vi "BlackBox.vi"() -> ()   [LabVIEW 2019]
uses:
  <vilib>/Simulation/Scripting/Companion Diagram/SimConfigNode/SimParams.ctl
  <vilib>/Simulation/Scripting/Companion Diagram/SimConfigNode/_simSolvers.ctl
  <vilib>/Simulation/Implementation/Shared/SIMSCR Execution Mode.ctl
  <vilib>/Simulation/Param Hierarchy/Typedefs/SIMPH Param Control Actions.ctl
  <vilib>/DAQmx/read.llb/DAQmx Read (Analog DBL 1Chan 1Samp).vi
  <vilib>/Simulation/Implementation/Shared/NILVSim_ParamChanged.vi
  <vilib>/Simulation/Implementation/Shared/NILVSIM_BeginStep.vi
  <vilib>/Simulation/Implementation/Shared/NILVSim_Manager.vi
  <vilib>/Utility/error.llb/Clear Errors.vi
  <vilib>/Simulation/Implementation/Shared/NILVSim_FinalizeModel.vi
  <vilib>/DAQmx/write.llb/DAQmx Write (Analog DBL 1Chan 1Samp).vi
  <vilib>/DAQmx/miscellaneous.llb/DAQmx Fill In Error Info.vi
  <vilib>/Simulation/Implementation/Shared/SIM Unbundle Sim Info.vi
  <vilib>/Simulation/Implementation/Shared/NILVSim_Initialize.vi
  <vilib>/Simulation/Utility/Implementation/NILVSim Get Time and IsAcceptedStep.vi
  <vilib>/Simulation/Implementation/Shared/SIMSH Read Queue.vi
  <vilib>/Simulation/Implementation/Shared/NILVSim_GetModelError.vi
  <vilib>/Simulation/Implementation/Shared/SIM Bundle Sim Info.vi
  <vilib>/Simulation/Implementation/XNodeFramework/SimXNode/SimX.xnode
  Industry 4-0 lab/Airheater Model subsystem.vi
  <vilib>/Simulation/Scripting/Companion Diagram/SimConfigNode/SimDog.xnode
  <vilib>/Simulation/Implementation/Shared/NI_SIM_Implementation.lvlib
panel:
  in  "stop":bool
  out "Temperature Chart":dbl(graph)
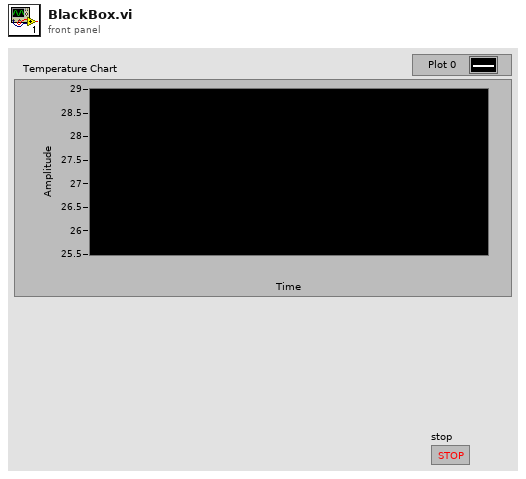
[diagram p1: front panel]
types:
  T1 = enum16{"Simulate to Completion", "Single Time-Step Simulation (Fixed Step Only)"}
  T2 = typedef "SIMSCR Execution Mode.ctl" = enum16{"Simulate to Completion", "Single Time-Step Simulation (Fixed Step Only)"}
  T3 = typedef "SIMPH Param Control Actions.ctl" = enum16{"get params", "set params"}
  T4 = cluster{"SIMSH Sim Time":dbl, "Operand2":dbl, "Multiplication 3":cluster{"Result":dbl}, "Integrator":cluster{"output":dbl}, "Multiplication 2":cluster{"Result":dbl}, "Summation 2":cluster{"Result":dbl}, "Transport Delay":cluster{"output":dbl}, "Summation":cluster{"Result":dbl}, "Multiplication":cluster{"Result":dbl}}
  T5 = typedef "SimParams.ctl" = cluster{"Initial Time (s)":dbl, "Final Time (s)":dbl, "Step Size (s)":dbl, "ODE Solver":T6, "Minimum Step Size (s)":dbl, "Maximum Step Size (s)":dbl, "Relative Tolerance":dbl, "Absolute Tolerance":dbl, "Software Timing":bool, "Initial Step Size (s)":dbl, "Automatic Fixed Step Size?":bool, "Automatic Discrete Step Size?":bool, "Discrete Step Size (s)":dbl, "Calculate using Time Step":bool, "Solver Wired?":bool, "Prev.Frm.Expected End":u64, "Prev.Frm.Actual End":u64, "Prev.Frm.Finished Late?":bool, "Prev.Iter.Expected End":u64, "Prev.Iter.Actual End":u64, "Prev.Iter.Finished Late?":bool, "Expected Iteration Start":u64, "Actual Iteration Start":u64, "Expected Frame Start":u64, "Actual Frame Start":u64, "Source Name":string, "Name":string, "Period":i64, "Deadline":i64, "Offset":i64, "Start":i64, "Priority":i32, "Timeout":i32, "Processor":i32, "Mode":enum32{"No Change", "Process missed periods, maintain original phase", "Discard missed periods, maintain original phase", "Process missed periods, ignore original phase", "Discard missed periods, ignore original phase"}, "Wakeup reason":enum32{"Normal", "Aborted", "Asynchronous wakeup", "Timing source error", "Timed loop error", "Timeout"}, "Error":errorcluster, "Source Type":string, "Secondary Source Type":string, "Global End Time":u64, "Global Start Time":u64, "Full Solver Reset":bool, "Execution Mode":T2, "Nan/Inf Check":bool, "Custom Solver Library":string, "Solver Is Variable":bool, "custom solver name":string, "Signal Collection Decimation":u32}
  T6 = typedef "_simSolvers.ctl" = enum16{"Runge-Kutta 1 (Euler)", "Runge-Kutta 2", "Runge-Kutta 3", "Runge-Kutta 4", "Runge-Kutta 23 (variable)", "Runge-Kutta 45 (variable)", "BDF (variable)", "Adams-Moulton (variable)", "Rosenbrock (variable)", "Discrete States Only", "SDIRK 4 (variable)", "Radau 5 (variable)", "Radau 9 (variable)", "Radau 13 (variable)", "Radau [Variable Order] (variable)", "Gear's Method (variable)", "Linearizer", "State Query", "Trim Eval", "Custom Solver"}
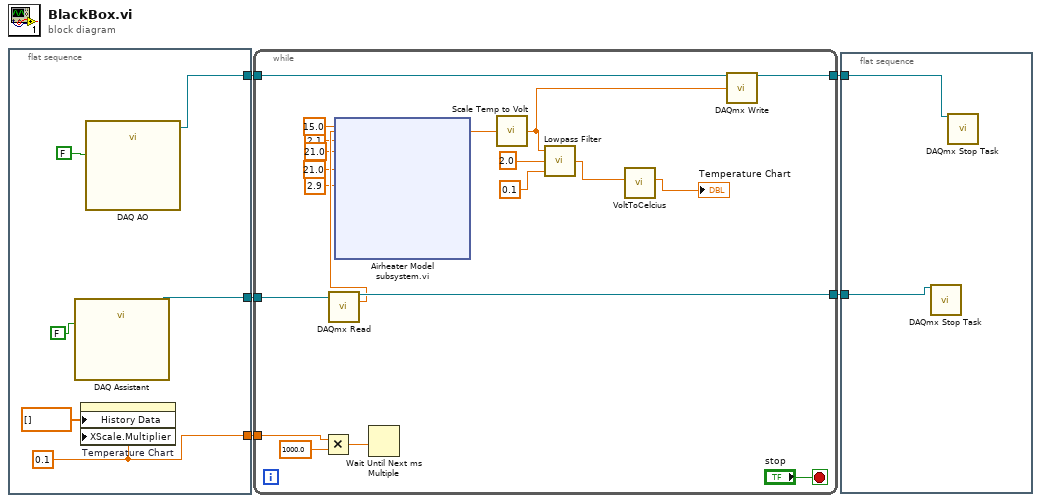
[diagram p0: block diagram]
diagram:
  n1 = flat-sequence {
    tunnel: [w10] -> w5
    tunnel: [w8] -> w3
    tunnel: [w6] -> w1
    frame #0 {
      w6 = 0.1 ("X Scale.Offset and Multiplier:Multiplier")
      n2 = call "DAQ Assistant"("stop (T)"=FALSE ("stop (F)")) -> ("task out"=w8:refnum<k21>)  [unwired: 16 in, 2 out]
      n3 = property on="Temperature Chart" class="WFChart (strict)"("History Data"=dbl[] [], "XScale.Multiplier"=w6) -> ()  [unwired: 2 in, 2 out]
      n4 = call "DAQ AO"("stop (T)"=FALSE) -> ("task out"=w10:refnum<k21>)  [unwired: 17 in, 1 out]
    }
  }
  n5 = while {
    tunnel: w5 -> [w28]
    tunnel: [w27] -> w4
    tunnel: w3 -> [w26]
    tunnel: [w25] -> w2
    tunnel: w1 -> [w21]
    stop <- "stop" stop-if-true
    n6 = Multiply(x=w21, y=1000.0) -> (x*y=w30:dbl)
    n7 = call-poly <vilib>:"DAQmx Read.vi"("task/channels in"=w26) -> ("task out"=w25:refnum<k21>, "data"=w20:dbl)  [unwired: 12 in, 1 out]
    n8 = xnode "Airheater Model subsystem.vi"("u [V]"=w20, "K [C/V]"=2.1, "T_enviroment [C]"=21.0, "T_initial [C]"=21.0, "Time constant [s]"=15.0, "Delay [s]"=2.9) -> ("T_out [C]"=w13:dbl)  [unwired: 2 in, 14 out]
    n9 = Wait Until Next ms Multiple(millisecond multiple=w30) -> ()  [unwired: 1 out]
    n10 = call "Scale Temp to Volt.vi"("Input Value (degC)"=w13) -> ("Output Value (V)"=w12:dbl)
    n11 = call "Lowpass Filter.vi"("Ts [s]"=0.1, "Tf [s]"=2.0, "Filter Input"=w12) -> ("Filter Output"=w14:dbl)
    n12 = call "VoltToCelcius.vi"("Voltage"=w14) -> ("Temperature[C]"=→"Temperature Chart":dbl)  [unwired: 10 in]
    n13 = call-poly <vilib>:"DAQmx Write.vi"("task/channels in"=w28, "data"=w12) -> ("task out"=w27:refnum<k21>)  [unwired: 11 in, 2 out]
  }
  n14 = flat-sequence {
    tunnel: w4 -> [w305]
    tunnel: w2 -> [w304]
    frame #0 {
      n15 = call <vilib>:"DAQmx Stop Task.vi"("task/channels in"=w304) -> ()  [unwired: 13 in, 2 out]
      n16 = call <vilib>:"DAQmx Stop Task.vi"("task/channels in"=w305) -> ()  [unwired: 13 in, 2 out]
    }
  }
